vi "Combined Status Monitor and Transient Capture (Array of Units Under Test).vi"(7 "Soft Trigger":bool, 9 "Post-Trigger Samples":i32, 10 "Pre-Trigger Samples":i32, 11 "List of INI Files":path[](array[path])) -> ()   [LabVIEW 2017]
uses:
  Status Monitor/Typedefs/Unit Under Test Status--Cluster.ctl
  SubVIs/Multi UUT GUI Commands--Enum.ctl
  SubVIs/Device Status and Index--Cluster.ctl
  Communications/Typedefs/DTACQ Module Carrier Status.ctl
  Communications/Typedefs/DTACQ Status--Enum.ctl
  Status Monitor/Status Monitor Library.lvlib
  Communications/Communications Library.lvlib
panel:
  in  "Graph All":bool
  in  "Stop Button":bool
  in  "Arm All":bool
  out "Device Status Messages":T1[](array[typedef])
  in  "error in":errorcluster
  in  "Previous Button":bool
  in  "Next Button":bool
  out "Selected UUT":string caption="Currently Selected Unit Under Test"
  in  "Graph":bool
  in  "Arm":bool
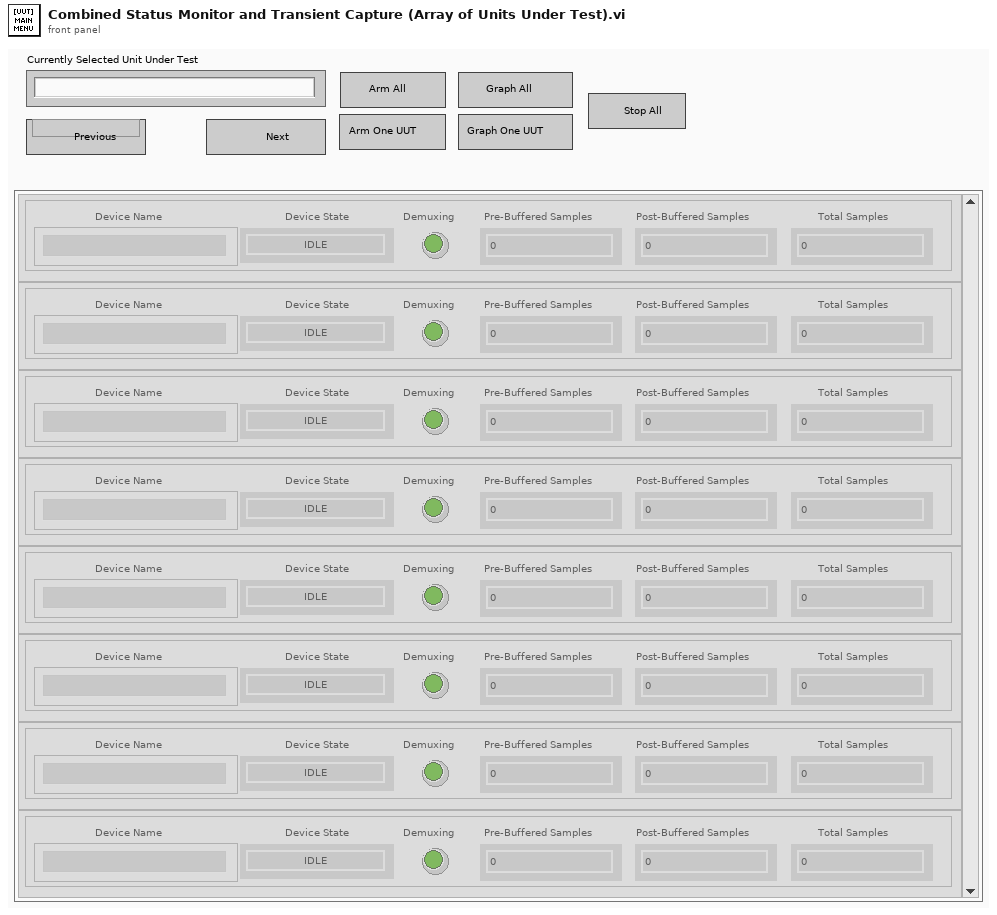
[diagram p1: front panel]
types:
  T1 = typedef "Status Monitor Library.lvlib/Unit Under Test Status--Cluster.ctl" = cluster{"Device State":enum16{"IDLE", "ARM", "RUN_PRE-TRIGGER", "RUN_POST-TRIGGER", "POST_PROCESS", "CLEANUP"}, "Pre-Buffered Samples":i32, "Post-Buffered Samples":i32, "Total Samples":i32, "Demuxing":bool, "Device Name":string}
  T2 = typedef "Device Status and Index--Cluster.ctl" = cluster{"Device Index":i32, "Module Carrier Status":T3}
  T3 = typedef "Communications Library.lvlib/DTACQ Module Carrier Status.ctl" = cluster{"DTACQ State":T4, "Pre-Trigger Samples":i32, "Post-Trigger Samples":i32, "Total Samples":i32, "Post Processing":bool}
  T4 = typedef "Communications Library.lvlib/DTACQ Status--Enum.ctl" = enum16{"IDLE", "ARM", "RUN_PRE-TRIGGER", "RUN_POST-TRIGGER", "POST_PROCESS", "CLEANUP"}
  T5 = typedef "Multi UUT GUI Commands--Enum.ctl" = enum16{"Shutdown", "Arm All", "Graph All", "Arm", "Graph", "Next", "Previous"}
  T6 = enum32{"Invalid", "Standard", "Closed", "Hidden", "Minimized", "Maximized"}
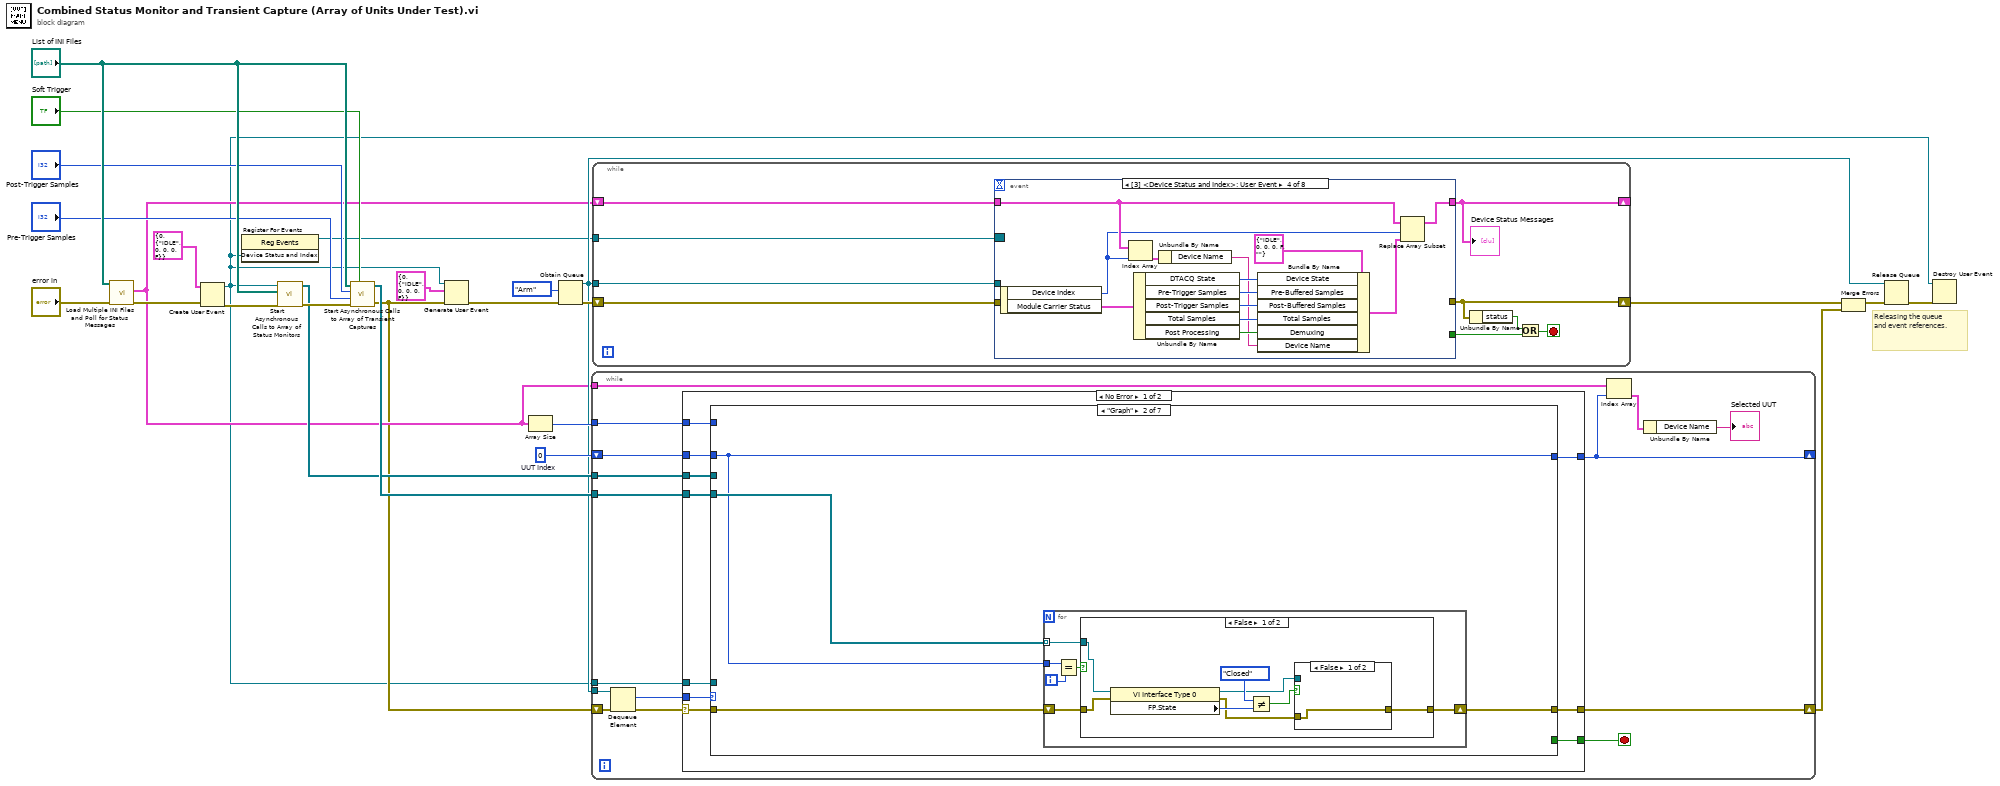
[diagram p0: block diagram]
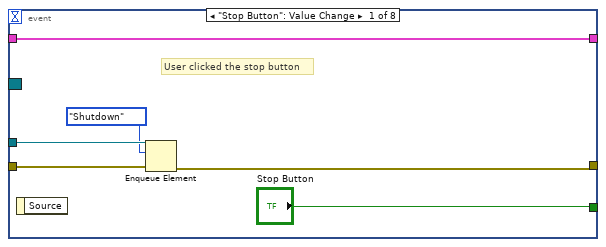
[diagram p2: hidden frame]
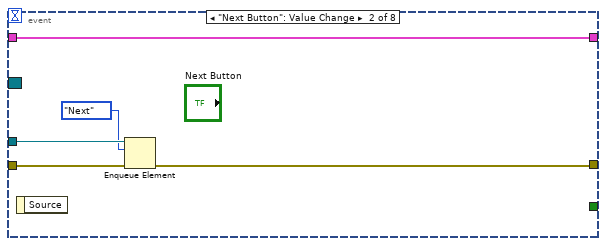
[diagram p3: hidden frame]
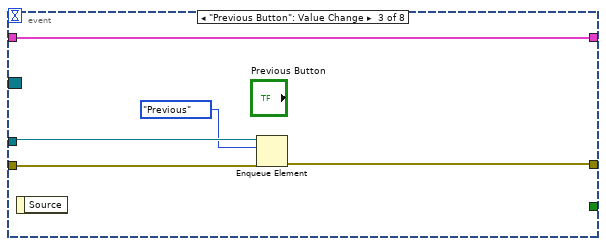
[diagram p4: hidden frame]
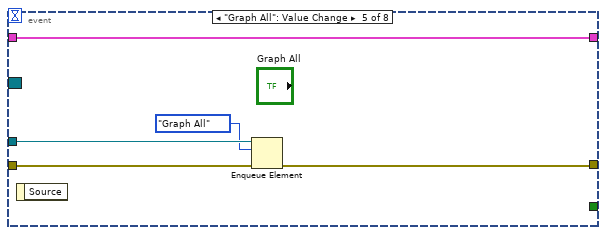
[diagram p5: hidden frame]
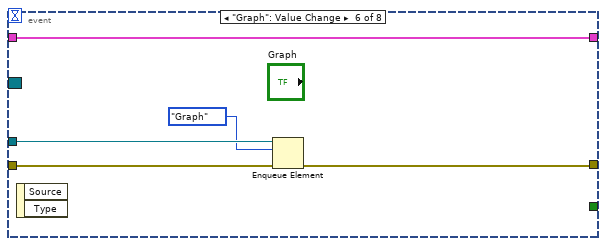
[diagram p6: hidden frame]
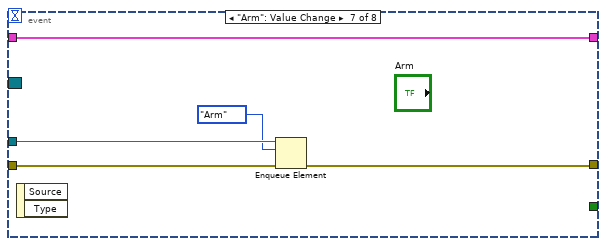
[diagram p7: hidden frame]
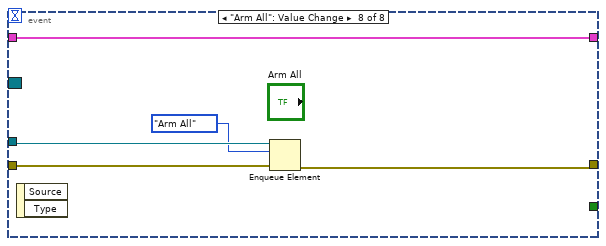
[diagram p8: hidden frame]
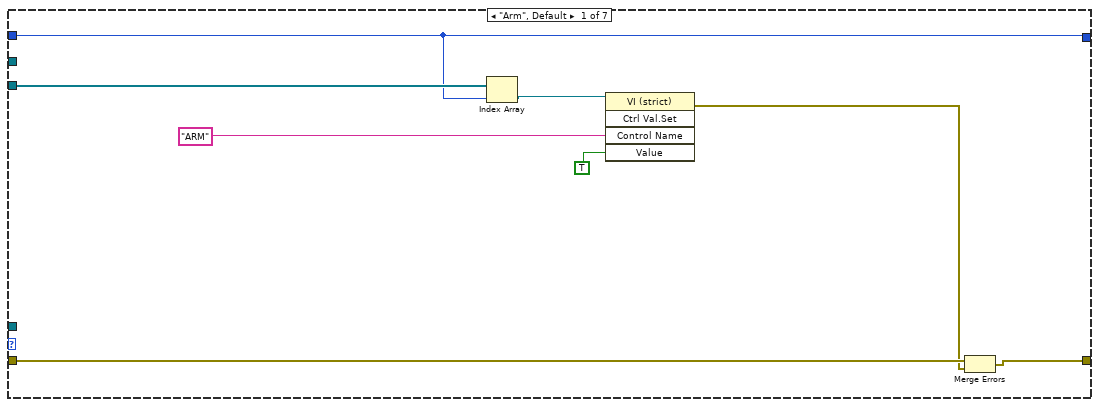
[diagram p9: hidden frame]
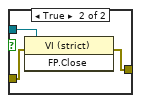
[diagram p10: hidden frame]
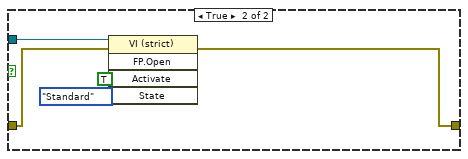
[diagram p11: hidden frame]
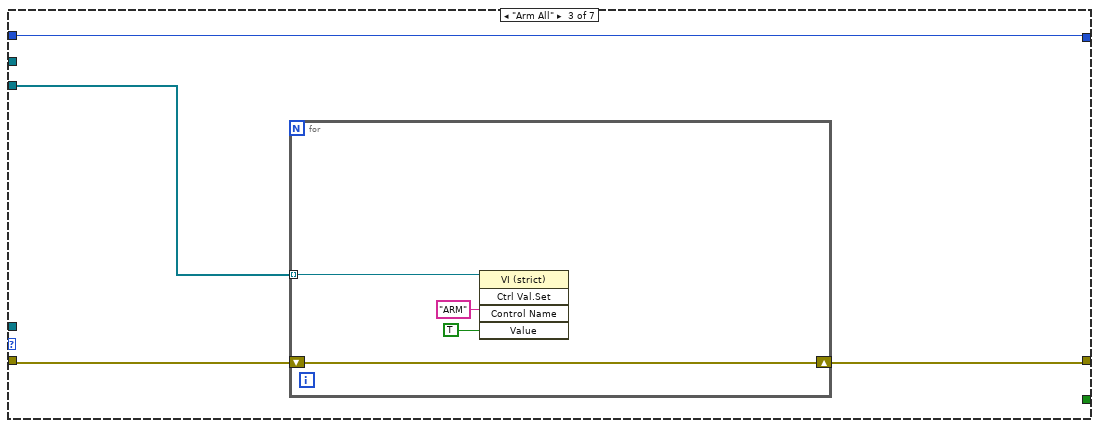
[diagram p12: hidden frame]
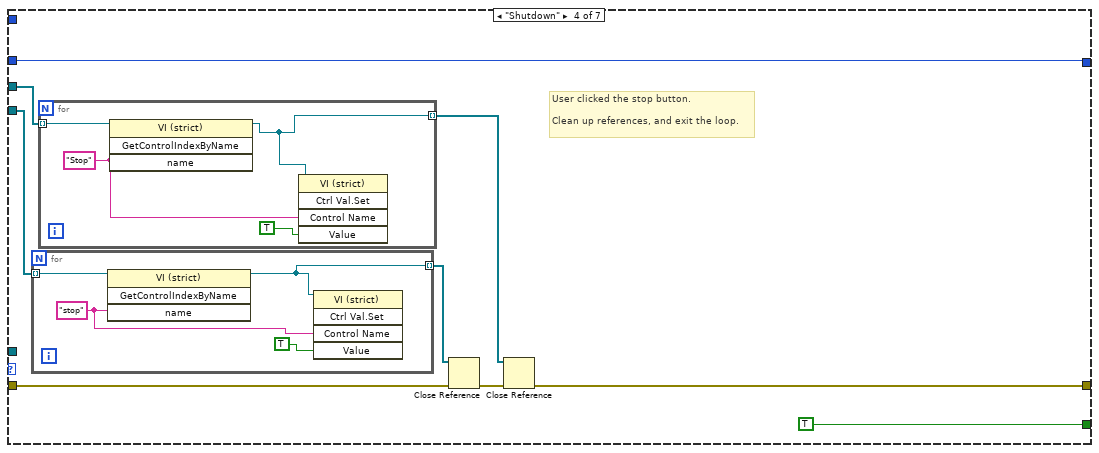
[diagram p13: hidden frame]
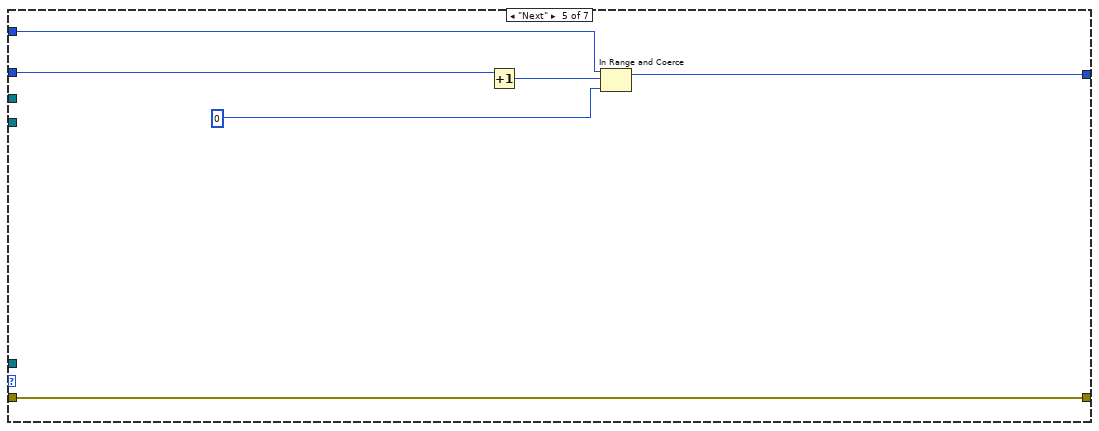
[diagram p14: hidden frame]
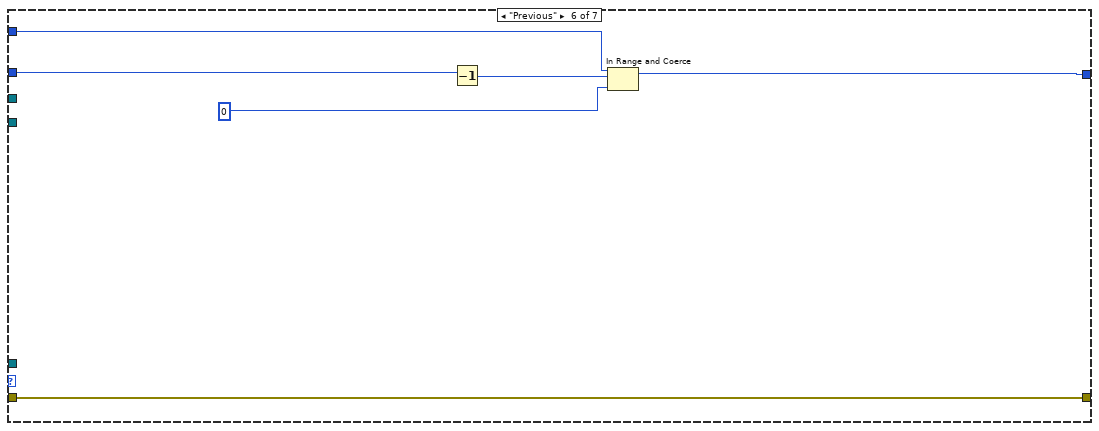
[diagram p15: hidden frame]
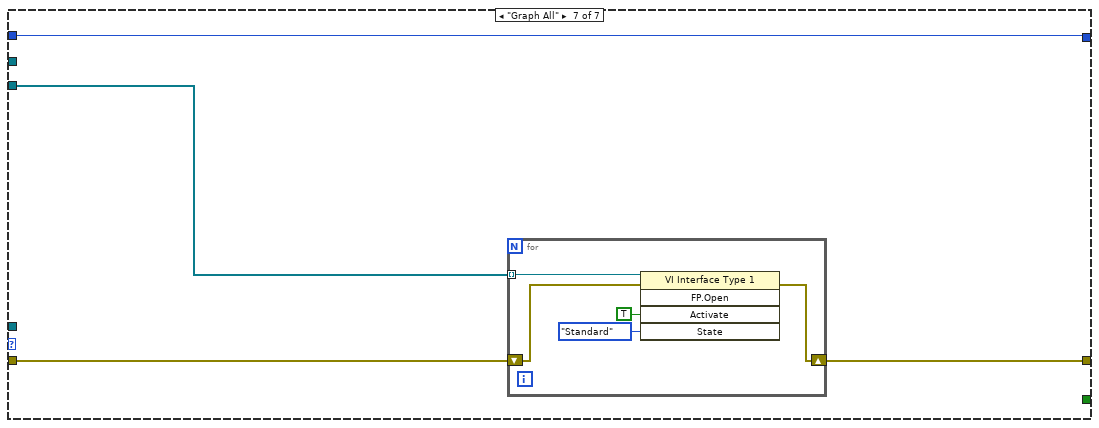
[diagram p16: hidden frame]
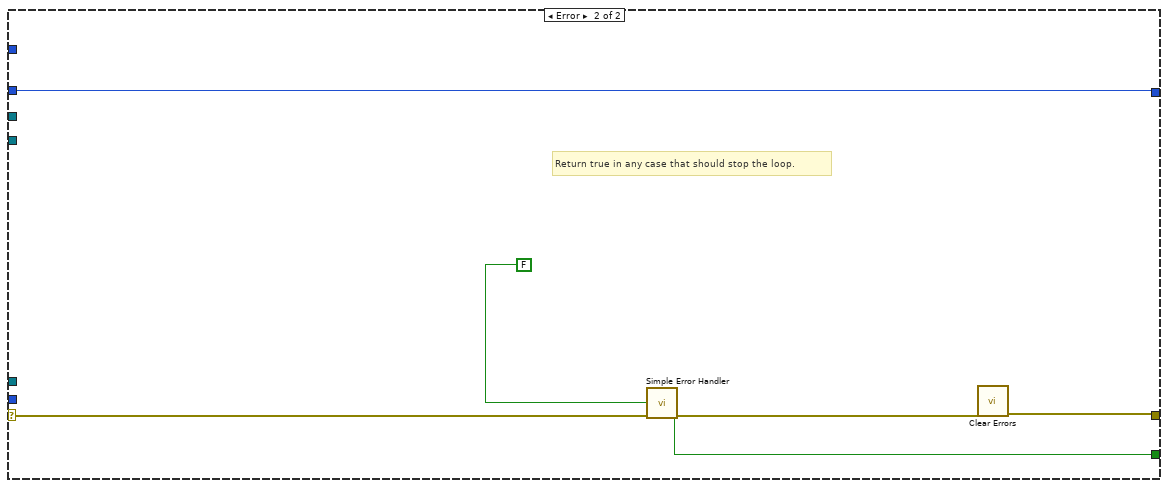
[diagram p17: hidden frame]
diagram:
  w25 = 0  # UUT Index
  # "Releasing the queue and event references."
  n1 = call "Load Multiple INI Files and Poll for Status Messages.vi"("error in"="error in", "List of INI Files"="List of INI Files") -> ("error out"=w23:errorcluster, "Device Status Messages"=w6:T1[])  [unwired: 7 in, 1 out]
  n2 = Create User Event(user event datatype=T2 {"Device Index"=0, "Module Carrier Status"={"DTACQ State"=enum."IDLE", "Pre-Trigger Samples"=0, "Post-Trigger Samples"=0, "Total Samples"=0, "Post Processing"=FALSE}} ("Device Status and Index"), error in=w23) -> (user event=w2:refnum<user-event>, error out=w21:errorcluster)
  n3 = register-events(w2) -> (reference out=w3:refnum<event-registration>)  [unwired: 2 in, 1 out]
  n4 = call "Start Asynchronous Calls to Array of Status Monitors.vi"("error in"=w21, "List of INI Files"="List of INI Files", "New Status Received - Event Reference"=w2) -> ("error out"=w18:errorcluster, "References to Instances"=w11:refnum<vi>[])  [unwired: 7 in]
  n5 = call "Start Asynchronous Calls to Array of Transient Captures.vi"("Soft Trigger"="Soft Trigger", "error in"=w18, "Pre-Trigger Samples"="Pre-Trigger Samples", "Post-Trigger Samples"="Post-Trigger Samples", "List of INI Files"="List of INI Files") -> ("error out"=w5:errorcluster, "References to Instances"=w13:refnum<vi>[])  [unwired: 5 in]
  n6 = Generate User Event(user event=w2, event data cluster=T2 {"Device Index"=0, "Module Carrier Status"={"DTACQ State"=enum."IDLE", "Pre-Trigger Samples"=0, "Post-Trigger Samples"=0, "Total Samples"=0, "Post Processing"=FALSE}} ("event data"), error in=w5) -> (error out=w4:errorcluster)  [unwired: 1 in, 1 out]
  n7 = Array Size(array=w6) -> (size(s)=w24:i32)
  n8 = Obtain Queue(element data type=Multi_UUT_GUI_Commands--Enum."Arm", error in (no error)=w4) -> (queue out=w8:refnum<queue>, error out=w9:errorcluster)  [unwired: 3 in, 1 out]
  n9 = while {
    tunnel: w8 -> [w41]
    shift-right: [w33] -> _
    shift-left: w25 -> [w36]
    tunnel: w24 -> [w35]
    tunnel: w6 -> [w34]
    shift-right: [w30] -> w12
    shift-left: w5 -> [w37]
    tunnel: w13 -> [w29]
    tunnel: w11 -> [w28]
    tunnel: w2 -> [w27]
    stop <- w38 stop-if-true
    n10 = Dequeue Element(queue=w41, error in (no error)=w37) -> (element=w39:T5, error out=w40:errorcluster)  [unwired: 1 in, 2 out]
    n11 = case shown="No Error" w40 {
      selector: w40 -> [w50 w136]
      tunnel: w39 -> [w51 _]
      tunnel: [w43 FALSE] -> w38
      tunnel: w36 -> [w49 w137]
      tunnel: [w48 w137] -> w33
      tunnel: w35 -> [w47 _]
      tunnel: [w46 w134] -> w30
      tunnel: w29 -> [w45 _]
      tunnel: w28 -> [w44 _]
      tunnel: w27 -> [w42 _]
      frame No Error {
        n12 = case shown="\"Graph\"" w51 {
          tunnel: w50 -> [w55 w61 w88 w102 w112 w118 w125]
          tunnel: w49 -> [w58 w62 w90 w103 w117 w122 w127]
          tunnel: [w58 w62 w90 w103 w113 w120 w127] -> w48
          tunnel: w47 -> [_ _ _ _ w115 w119 _]
          tunnel: [w52 w60 w89 w100 w112 w118 w124] -> w46
          tunnel: w45 -> [w59 w63 w87 w98 _ _ w126]
          tunnel: w44 -> [_ _ _ w95 _ _ _]
          tunnel: [_ _ _ TRUE _ _ _] -> w43
          tunnel: w42 -> [_ _ _ _ _ _ _]
          frame "Arm", Default {
            n13 = Index Array(array=w59, index=w58) -> (element=w56:refnum<vi>)
            n14 = invoke class="VI (strict)" method="Ctrl Val.Set"(reference=w56, "Control Name"="ARM", "Value"=TRUE) -> (error out=w54:errorcluster)  [unwired: 2 in, 4 out]
            n15 = Merge Errors(w55, w54) -> (w52:errorcluster)
          }
          frame "Graph" {
            n16 = for {
              tunnel: w63 -> [w69] mode=indexing
              tunnel: w62 -> [w68]
              shift-right: [w64] -> w60
              shift-left: w61 -> [w65]
              i -> [w67]
              n17 = Equal?(x=w68, y=w67) -> (x = y?=w66:bool)
              n18 = case shown="False" w66 {
                tunnel: w69 -> [w76 w84]
                tunnel: w65 -> [w77 w83]
                tunnel: [w70 w82] -> w64
                frame False {
                  n19 = property class="VI Interface Type 0"(reference=w76, error in=w77) -> (reference out=w72:refnum<vi>, error out=w71:errorcluster, "FP.State"=w74:T6)
                  n20 = Not Equal?(x=T6."Closed", y=w74) -> (x != y?=w73:bool)
                  n21 = case shown="False" w73 {
                    tunnel: w72 -> [_ w81]
                    tunnel: w71 -> [w78 w80]
                    tunnel: [w78 w79] -> w70
                    frame False {
                    }
                    frame True {
                      n22 = invoke class="VI (strict)" method="FP.Close"(reference=w81, error in=w80) -> (error out=w79:errorcluster)  [unwired: 1 in, 2 out]
                    }
                  }
                }
                frame True {
                  n23 = invoke class="VI (strict)" method="FP.Open"(reference=w84, error in=w83, "Activate"=TRUE ("Activate?"), "State"=T6."Standard") -> (error out=w82:errorcluster)  [unwired: 1 in, 4 out]
                }
              }
            }
          }
          frame "Arm All" {
            n24 = for {
              shift-right: [w91] -> w89
              shift-left: w88 -> [w91]
              tunnel: w87 -> [w93] mode=indexing
              n25 = invoke class="VI (strict)" method="Ctrl Val.Set"(reference=w93, "Control Name"="ARM", "Value"=TRUE) -> ()  [unwired: 2 in, 5 out]
            }
          }
          frame "Shutdown" {
            # "User clicked the stop button.\n\nClean up references, and exit the loop."
            n26 = for {
              tunnel: w98 -> [w111] mode=indexing
              tunnel: [w108] -> w97 mode=indexing
              w110 = "stop"
              n27 = invoke class="VI (strict)" method="GetControlIndexByName"(reference=w111, "name"=w110) -> (reference out=w108:refnum<vi>)  [unwired: 2 in, 3 out]
              n28 = invoke class="VI (strict)" method="Ctrl Val.Set"(reference=w108, "Control Name"=w110, "Value"=TRUE) -> ()  [unwired: 2 in, 5 out]
            }
            n29 = for {
              tunnel: w95 -> [w107] mode=indexing
              tunnel: [w106] -> w96 mode=indexing
              w105 = "Stop"
              n30 = invoke class="VI (strict)" method="GetControlIndexByName"(reference=w107, "name"=w105) -> (reference out=w106:refnum<vi>)  [unwired: 2 in, 3 out]
              n31 = invoke class="VI (strict)" method="Ctrl Val.Set"(reference=w106, "Control Name"=w105, "Value"=TRUE) -> ()  [unwired: 2 in, 5 out]
            }
            n32 = Close Reference(reference=w97, error in (no error)=w102) -> (error out=w101:errorcluster)
            n33 = Close Reference(reference=w96, error in (no error)=w101) -> (error out=w100:errorcluster)
          }
          frame "Next" {
            n34 = Increment(x=w117) -> (x+1=w116:i32)
            n35 = In Range and Coerce(upper limit=w115, x=w116, lower limit=0) -> (coerced(x)=w113:i32)  [unwired: 1 out]
          }
          frame "Previous" {
            n36 = Decrement(x=w122) -> (x-1=w121:i32)
            n37 = In Range and Coerce(upper limit=w119, x=w121, lower limit=0) -> (coerced(x)=w120:i32)  [unwired: 1 out]
          }
          frame "Graph All" {
            n38 = for {
              tunnel: w126 -> [w132] mode=indexing
              shift-right: [w128] -> w124
              shift-left: w125 -> [w129]
              n39 = invoke class="VI Interface Type 1" method="FP.Open"(reference=w132, error in=w129, "Activate"=TRUE ("Activate?"), "State"=T6."Standard") -> (error out=w128:errorcluster)  [unwired: 1 in, 4 out]
            }
          }
        }
      }
      frame Error {
        # "Return true in any case that should stop the loop."
        n40 = call <vilib>:"Simple Error Handler.vi"("error in (no error)"=w136) -> ("error out"=w135:errorcluster)  [unwired: 4 in, 4 out]
        n41 = call <vilib>:"Clear Errors.vi"("error in (no error)"=w135) -> ("error out"=w134:errorcluster)  [unwired: 5 in, 1 out]
      }
    }
    n42 = Index Array(array=w34, index=w33) -> (element=w32:T1)
    n43 = Unbundle By Name(w32) -> ("Device Name"=→"Selected UUT":string)
  }
  n44 = while {
    shift-right: [w142] -> w19
    shift-left: w9 -> [w145]
    tunnel: w8 -> [w146]
    tunnel: w3 -> [w140]
    shift-right: [w138] -> _
    shift-left: w6 -> [w139]
    stop <- w143 stop-if-true
    n45 = event shown="[3] <Device Status and Index>: User Event" {
      selector: w140 -> [_ _ _ _ _ _ _ _]
      dyn-events: _ -> [_ _ _ _ _ _ _ _]
      timeout: _ -> [_ _ _ _ _ _ _ _]
      tunnel: w146 -> [w149 w156 w160 _ w177 w182 w187 w192]
      tunnel: w145 -> [w150 w157 w161 _ w179 w184 w189 w194]
      tunnel: [w147 w154 w159 _ w178 w183 w188 w193] -> w142
      tunnel: ["Stop Button" _ _ _ _ _ _ _] -> w144
      tunnel: w139 -> [w152 w153 w162 w166 w180 w185 w190 w195]
      tunnel: [w152 w153 w162 w167 w180 w185 w190 w195] -> w138
      event "Stop Button": Value Change {
        # "User clicked the stop button"
        n46 = event-data() -> ()  [unwired: 1 in, 1 out]
        n47 = Enqueue Element(queue=w149, element=Multi_UUT_GUI_Commands--Enum."Shutdown", error in (no error)=w150) -> (error out=w147:errorcluster)  [unwired: 1 in, 2 out]
      }
      event "Next Button": Value Change {
        n48 = event-data() -> ()  [unwired: 1 in, 1 out]
        n49 = Enqueue Element(queue=w156, element=Multi_UUT_GUI_Commands--Enum."Next", error in (no error)=w157) -> (error out=w154:errorcluster)  [unwired: 1 in, 2 out]
      }
      event "Previous Button": Value Change {
        n50 = event-data() -> ()  [unwired: 1 in, 1 out]
        n51 = Enqueue Element(queue=w160, element=Multi_UUT_GUI_Commands--Enum."Previous", error in (no error)=w161) -> (error out=w159:errorcluster)  [unwired: 1 in, 2 out]
      }
      event User Event {
        n52 = event-data() -> ("Device Index"=w165:i32, "Module Carrier Status"=w174:T3)  [unwired: 1 in]
        n53 = Index Array(array=w166, index=w165) -> (element=w164:T1)
        n54 = Unbundle By Name(w174) -> ("DTACQ State"=w173:T4, "Pre-Trigger Samples"=w172:i32, "Post-Trigger Samples"=w171:i32, "Total Samples"=w170:i32, "Post Processing"=w169:bool)
        n55 = Unbundle By Name(w164) -> ("Device Name"=w163:string)
        n56 = Bundle By Name(cluster=T1 {"Device State"=enum."IDLE", "Pre-Buffered Samples"=0, "Post-Buffered Samples"=0, "Total Samples"=0, "Demuxing"=FALSE, "Device Name"=""} ("Status Cluster"), "Device State"=w173, "Pre-Buffered Samples"=w172, "Post-Buffered Samples"=w171, "Total Samples"=w170, "Demuxing"=w169, "Device Name"=w163) -> (w168:T1)
        n57 = Replace Array Subset(array=w166, new element=w168, index=w165) -> (w167:T1[])
      }
      event "Graph All": Value Change {
        n58 = event-data() -> ()  [unwired: 1 in, 1 out]
        n59 = Enqueue Element(queue=w177, element=Multi_UUT_GUI_Commands--Enum."Graph All", error in (no error)=w179) -> (error out=w178:errorcluster)  [unwired: 1 in, 2 out]
      }
      event "Graph": Value Change {
        n60 = event-data() -> ()  [unwired: 1 in, 2 out]
        n61 = Enqueue Element(queue=w182, element=Multi_UUT_GUI_Commands--Enum."Graph", error in (no error)=w184) -> (error out=w183:errorcluster)  [unwired: 1 in, 2 out]
      }
      event "Arm": Value Change {
        n62 = event-data() -> ()  [unwired: 1 in, 2 out]
        n63 = Enqueue Element(queue=w187, element=Multi_UUT_GUI_Commands--Enum."Arm", error in (no error)=w189) -> (error out=w188:errorcluster)  [unwired: 1 in, 2 out]
      }
      event "Arm All": Value Change {
        n64 = event-data() -> ()  [unwired: 1 in, 2 out]
        n65 = Enqueue Element(queue=w192, element=Multi_UUT_GUI_Commands--Enum."Arm All", error in (no error)=w194) -> (error out=w193:errorcluster)  [unwired: 1 in, 2 out]
      }
    }
    "Device Status Messages" <- w138
    n66 = Unbundle By Name(w142) -> ("status"=w141:bool)
    n67 = Or(x=w141, y=w144) -> (x .or. y?=w143:bool)
  }
  n68 = Merge Errors(w19, w12) -> (w20:errorcluster)
  n69 = Release Queue(queue=w8, error in (no error)=w20) -> (error out=w10:errorcluster)  [unwired: 1 in, 2 out]
  n70 = Destroy User Event(user event=w2, error in=w10) -> ()  [unwired: 1 out]
